vi "Top Level State Machine.vi"(8 "error in":errorcluster, 9 "Buses":T2[](array[typedef])=[{"Devices"=[{"Number of Channels"=1, "Device Alias"="", "Device Icon Name"=[]}], "Pin Information"={"List of IO Names"=["sbRIO-9651 Socket\\PMOD1_Pin4_out", "sbRIO-9651 Socket\\PMOD1_Pin3_in", "sbRIO-9651 Socket\\PMOD1_Pin2_out", "sbRIO-9651 Socket\\PMOD1_Pin1_out"], "List of Enable Lines"=["sbRIO-9651 Socket\\PMOD1_Pin4_enable", "sbRIO-9651 Socket\\PMOD1_Pin3_enable", "sbRIO-9651 Socket\\PMOD1_Pin2_enable", "sbRIO-9651 Socket\\PMOD1_Pin1_enable"]}, "Replacement VI for DLU"=path "E:/Documents/Projects/SPIAPI/Scripting Code  with State Machine 01_16_15 - Integrating with GUI/Test/Replacement.vi"}], 10 "Input Paths":T1={"Golden Template Directory"=path "E:/Documents/Projects/SPIAPI/Scripting Code  with State Machine 01_16_15 - Integrating with GUI/IONode", "Destination Directory"=path "E:/Documents/Projects/SPIAPI/Scripting Code  with State Machine 01_16_15 - Integrating with GUI/Test", "Destination Project"=path "E:/Documents/Projects/SPIAPI/Scripting Code  with State Machine 01_16_15 - Integrating with GUI/Test/Test.lvproj", "Destination VI"=path "E:/Documents/Projects/SPIAPI/Scripting Code  with State Machine 01_16_15 - Integrating with GUI/Test/TestVI.VI"}) -> (0 "error out":errorcluster)   [LabVIEW 2014, in "Initialization and IO Node Scripting.lvlib"]
uses:
  Initialization and IO Node Scripting.lvlib
  Scripting States.ctl
  Controls/Bus Information.ctl
  Controls/Device Information.ctl
  Controls/Pin Information.ctl
  Controls/Input Paths.ctl
  Controls/Values for Naming.ctl
  System.Windows.Forms
panel:
  out "Elapsed Time":dbl format="%<%H:%M:%S>t"
  in  "ProgressBar":refnum<k24>(container)
  in  "?":T5
  out "Status":string
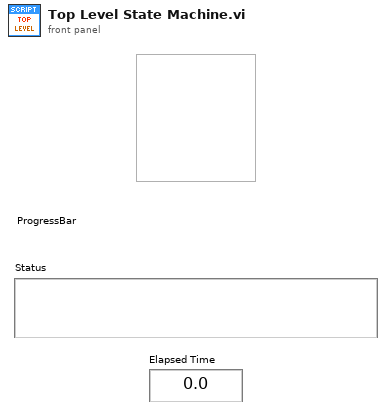
[diagram p1: front panel]
types:
  T1 = typedef "Input Paths.ctl" = cluster{"Golden Template Directory":path, "Destination Directory":path, "Destination Project":path, "Destination VI":path}
  T2 = typedef "Initialization and IO Node Scripting.lvlib/Bus Information.ctl" = cluster{"Devices":T3[], "Pin Information":T4, "Replacement VI for DLU":path}
  T3 = typedef "Device Information.ctl" = cluster{"Number of Channels":i32, "Device Alias":string, "Device Icon Name":string[]}
  T4 = typedef "Pin Information.ctl" = cluster{"List of IO Names":string[], "List of Enable Lines":string[]}
  T5 = typedef "Scripting States.ctl" = enum16{"Initialize", "Modify Dequeue Commands", "Modify Enqueue Data", "Create Project FIFOs", "Create and Place IO Nodes", "Update Node Count in Engine", "Expand FIFO Type Def", "Populate FIFO Names in Engine", "Modify I/O Pin Names", "Modify I/O Pin Enable", "Replace DLU", "Place SPI Engine", "Buses Complete Check", "End"}
  T6 = typedef "Initialization and IO Node Scripting.lvlib/Values for Naming.ctl" = cluster{"Bus Number":i32, "Device Number":i32, "Channel Number":i32}
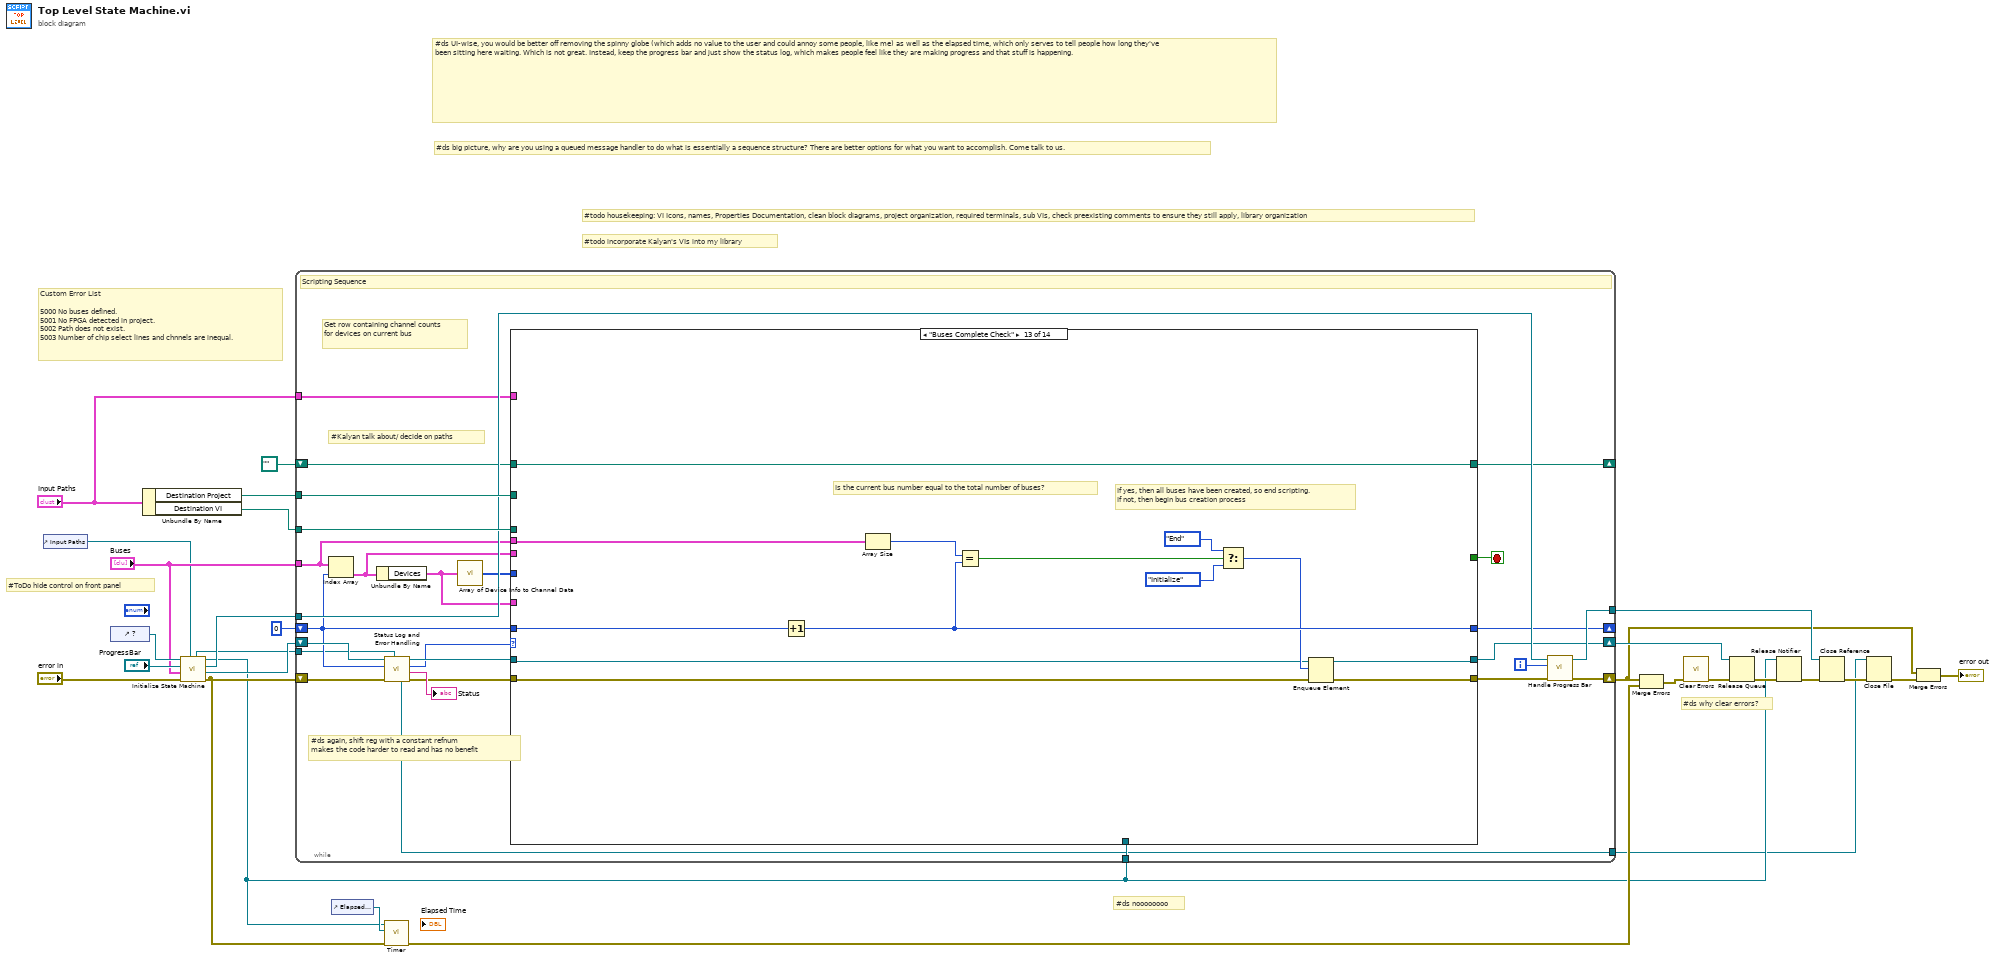
[diagram p0: block diagram]
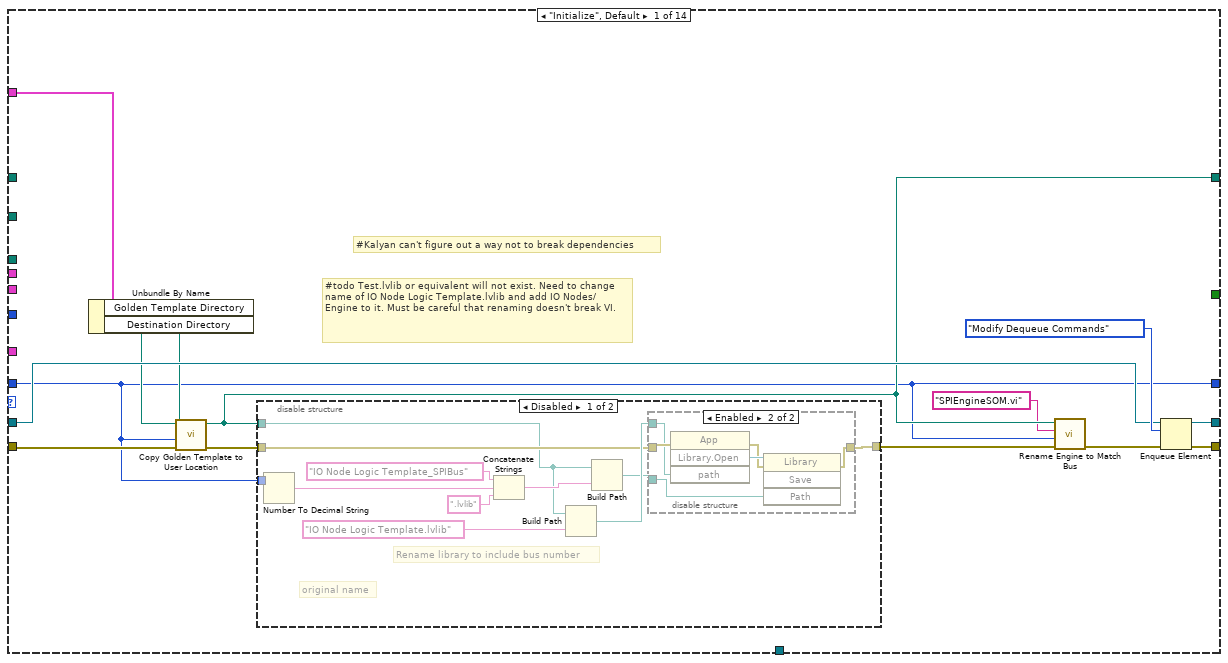
[diagram p2: hidden frame]
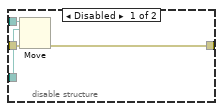
[diagram p3: hidden frame]
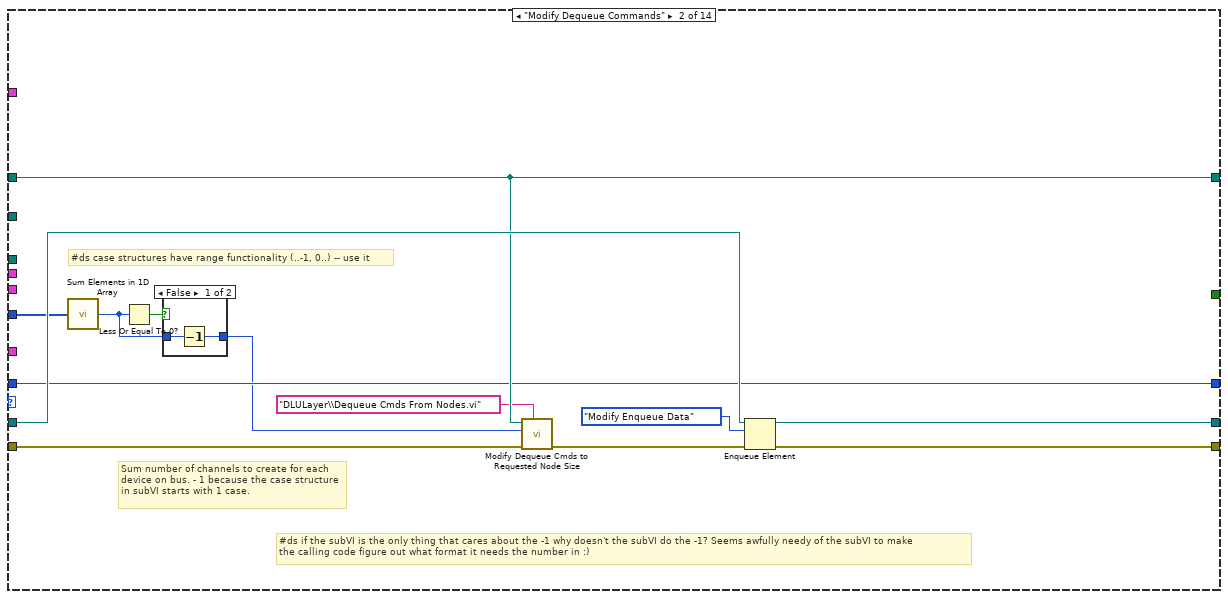
[diagram p5: hidden frame]
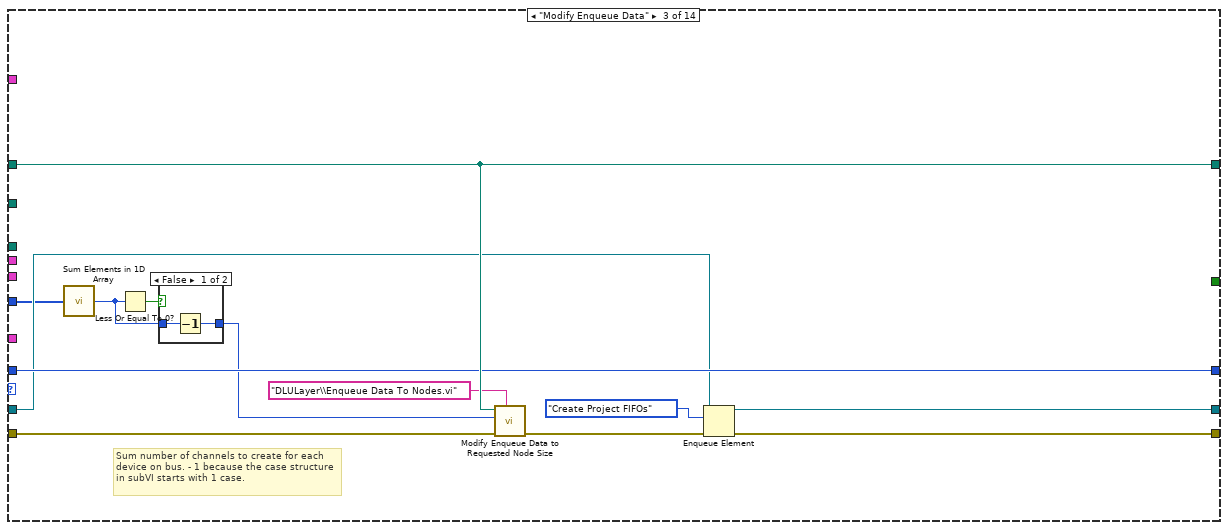
[diagram p7: hidden frame]
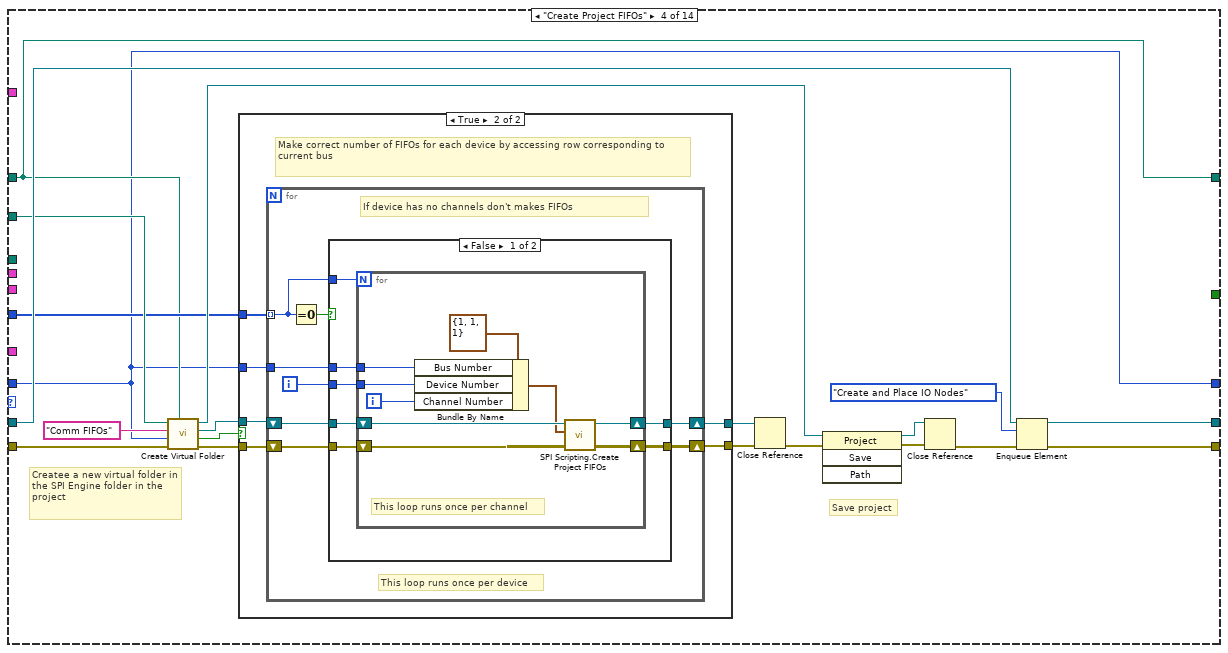
[diagram p9: hidden frame]
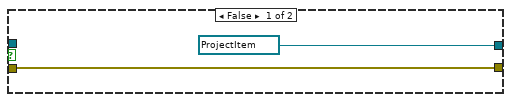
[diagram p10: hidden frame]
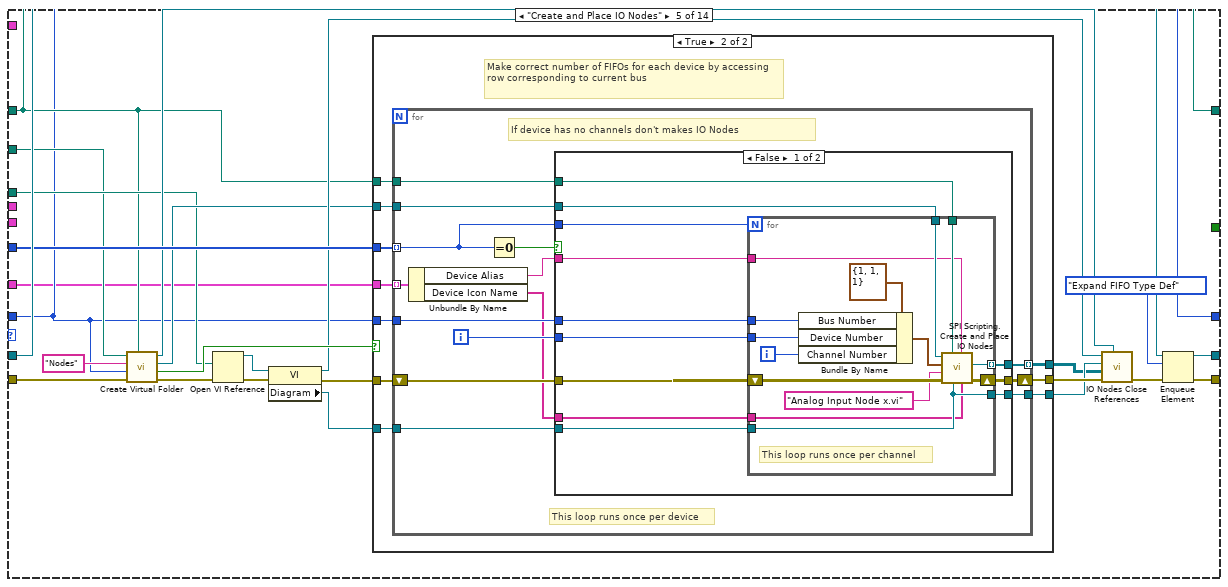
[diagram p12: hidden frame]
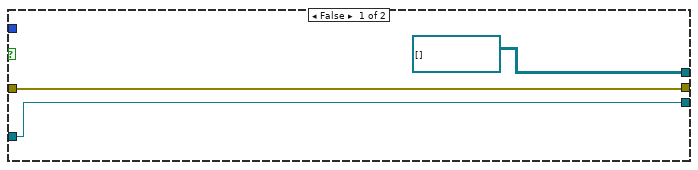
[diagram p13: hidden frame]
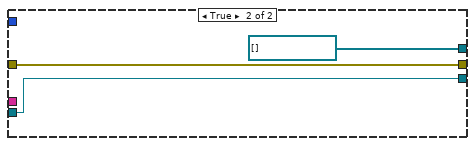
[diagram p14: hidden frame]
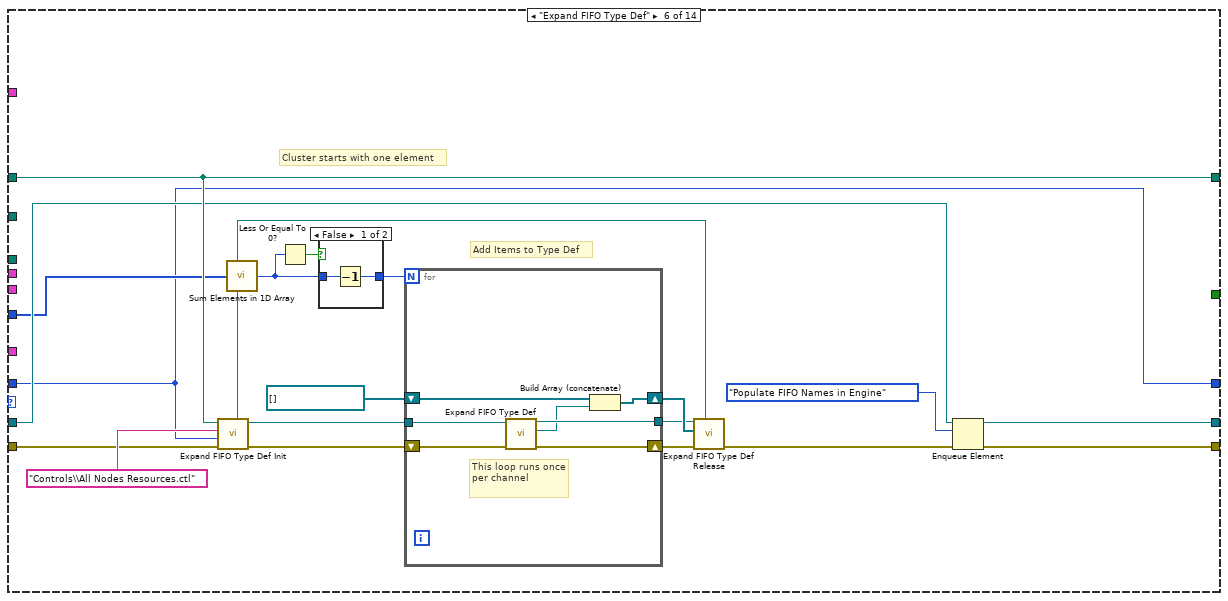
[diagram p15: hidden frame]
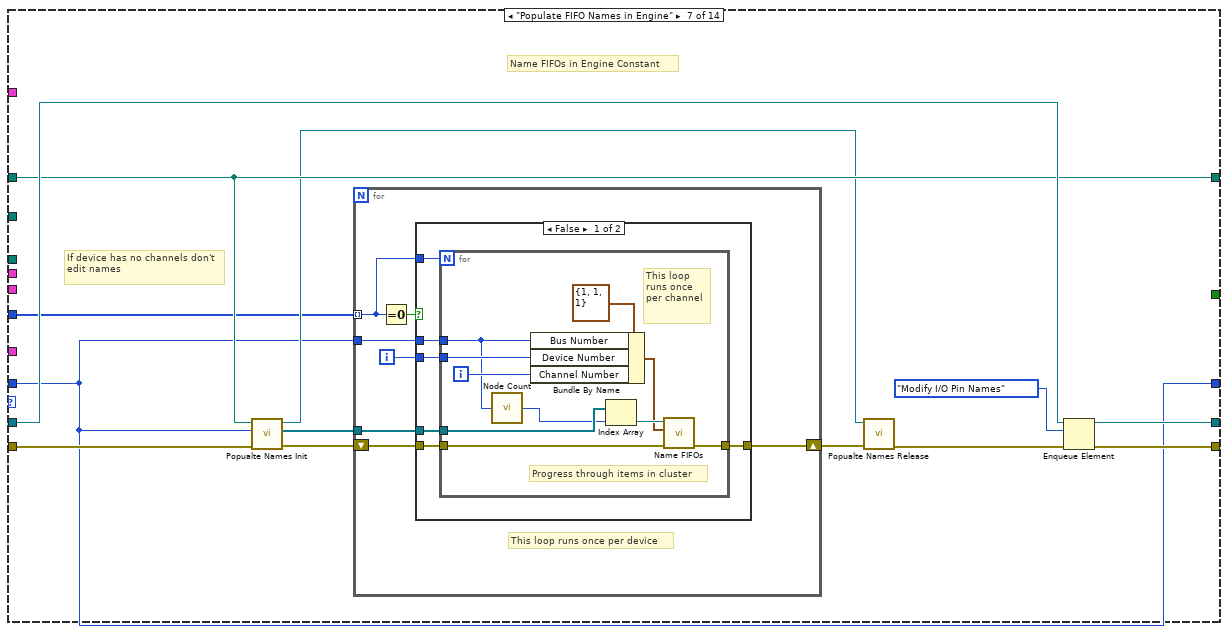
[diagram p17: hidden frame]
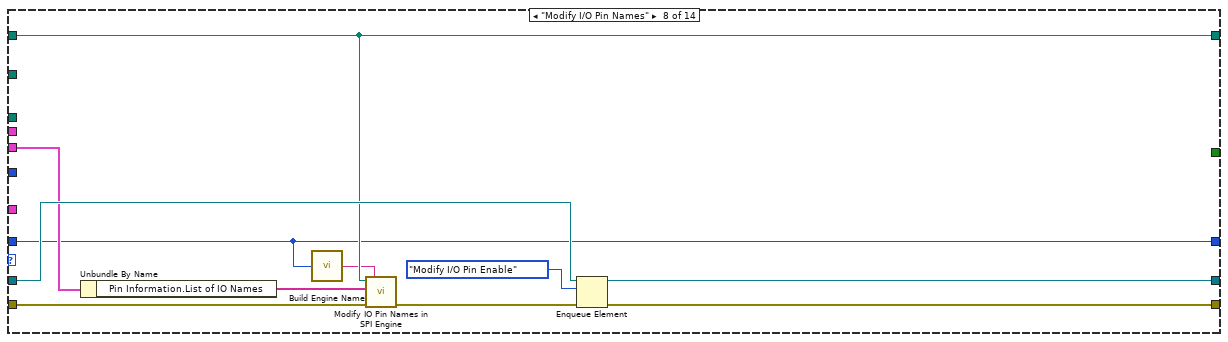
[diagram p19: hidden frame]
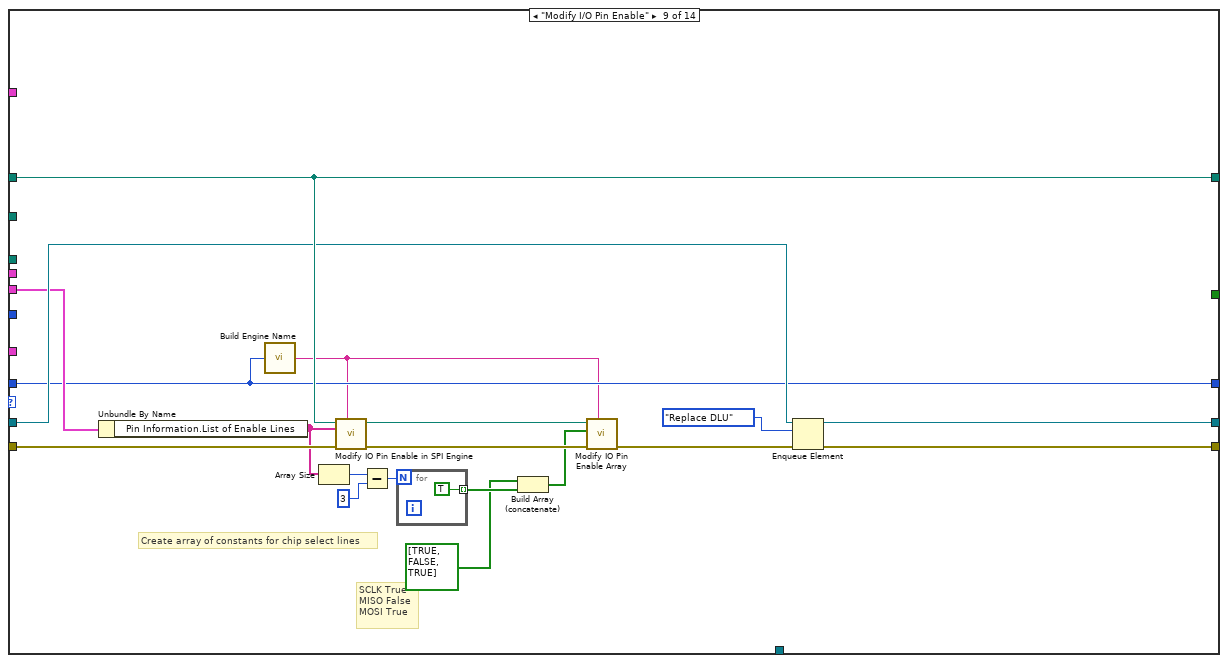
[diagram p20: hidden frame]
diagram:
  # "#ds big picture, why are you using a queued message handler to do what is essentially a sequence structure? There are better options for what you want to accomplish. Come talk to us."
  # "#ds why clear errors?"
  # "#ds noooooooo"
  # "#ds UI-wise, you would be better off removing the spinny globe (which adds no value to the user and could annoy some people, like me) as well as the elapsed time, which only serves to tell people how long they've been sitting here waiting. Which is not great. Instead, keep the progress bar and just show the status log, which makes people feel like they are making progress and that stuff is happening."
  # "Custom Error List\n\n5000 No buses defined.\n5001 No FPGA detected in project.\n5002 Path does not exist.\n5003 Number of chip select lines and chnnels are inequal."
  # "#todo incorporate Kalyan's VIs into my library"
  # "#todo housekeeping: VI Icons, names, Properties Documentation, clean block diagrams, project organization, required terminals, sub VIs, check preexisting comments to ensure they still apply, library organization"
  # "#ToDo hide control on front panel"
  n1 = control-ref of="Input Paths"() -> (w1:refnum<vi>)
  n2 = control-ref of="?"() -> (w16:refnum<vi>)
  n3 = Unbundle By Name("Input Paths") -> ("Destination Project"=w13:path, "Destination VI"=w12:path)
  n4 = call "Initialize State Machine.vi"("Input Paths Refnum"=w1, "error in (no error)"="error in", "Bus Info"="Buses", "ProgressBar in"="ProgressBar", "Enum Refnum"=w16) -> ("error out"=w26:errorcluster, "queue out"=w28:refnum<queue>, "ProgressBar out"=w22:refnum<k24>, "Notifier out"=w15:refnum<notifier>, "Status Log"=w3:refnum<file>)  [unwired: 2 in]
  n5 = while {
    shift-right: [w45] -> w9
    shift-left: w26 -> [w35]
    shift-right: [w46] -> w20
    shift-left: w28 -> [w37]
    tunnel: [w54] -> w23
    tunnel: w22 -> [w50]
    tunnel: w13 -> [w52]
    tunnel: w12 -> [w53]
    shift-right: [w49] -> _
    shift-left: 0 ("Number of SPI Buses") -> [w36]
    shift-right: [w48] -> _
    shift-left: path "" ("Curent Bus Path") -> [w47]
    tunnel: w15 -> [w43]
    tunnel: "Buses" -> [w42]
    tunnel: "Input Paths" -> [w40]
    tunnel: w3 -> [w30]
    tunnel: [w29] -> w2
    i -> [w51]
    stop <- w44 stop-if-true
    # "#ds again, shift reg with a constant refnum\nmakes the code harder to read and has no benefit"
    # "#Kalyan talk about/ decide on paths"
    # "Get row containing channel counts for devices on current bus"
    # "Scripting Sequence"
    n6 = Index Array(array=w42, index=w36) -> (element=w41:T2)
    n7 = Unbundle By Name(w41) -> ("Devices"=w38:T3[])
    n8 = call "Status Log and Error Handling.vi"("Status Log"=w30, "error in"=w35, "Current Bus Number"=w36, "Queue in"=w37) -> ("error out"=w31:errorcluster, "Current Status"=→"Status":string, "Next State"=w33:T5, "Queue out"=w34:refnum<queue>, "Status Log"=w29:refnum<file>)  [unwired: 3 in]
    n9 = call "Array of Device Info to Channel Data.vi"("Array of Devices"=w38) -> ("Device Channels"=w39:i32[])
    n10 = case shown="\"Buses Complete Check\"" w33 {
      tunnel: [w61 w92 w119 w142 w201 w268 w300 w335 w354 w365 w382 w399 w411 w422] -> w55
      tunnel: [w69 w104 w120 w143 w202 w267 w301 w336 w355 w366 w381 w400 w412 w427] -> w46
      tunnel: w31 -> [w67 w99 w115 w138 w194 w271 w291 w331 w352 w363 w377 w394 w413 w423]
      tunnel: w34 -> [w66 w102 w112 w140 w199 w266 w298 w333 w347 w364 w375 w396 w414 w427]
      tunnel: w47 -> [_ w100 w117 w125 w180 w270 w295 w330 w349 w361 w376 w391 w410 w430]
      tunnel: w52 -> [_ _ _ w137 w182 _ _ _ _ _ _ w384 _ _]
      tunnel: w53 -> [_ _ _ _ w183 _ _ _ _ _ _ w397 _ _]
      tunnel: w39 -> [_ w96 w109 w126 w198 w260 w290 _ _ _ w380 _ _ _]
      tunnel: w36 -> [w57 w98 w114 w124 w179 w259 w289 w327 w338 w360 w372 w392 w421 w431]
      tunnel: [w57 w98 w114 w124 w179 w259 w289 w327 w338 w360 w372 w392 w419 w431] -> w49
      tunnel: w42 -> [_ _ _ _ _ _ _ _ _ _ _ _ w418 _]
      tunnel: [w63 w100 w117 w125 w180 w270 w295 w330 w349 w361 w376 w391 w410 w430] -> w48
      tunnel: [_ _ _ _ _ _ _ _ _ _ _ _ _ TRUE] -> w44
      tunnel: w43 -> [_ _ _ _ _ _ _ _ _ _ _ _ _ w426]
      tunnel: w41 -> [_ _ _ _ _ _ _ w329 w343 w359 _ _ _ _]
      tunnel: w40 -> [w60 _ _ _ _ _ _ _ _ _ _ _ _ _]
      tunnel: w38 -> [_ _ _ _ w178 _ _ _ _ _ _ _ _ _]
      frame "Initialize", Default {
        # "#Kalyan can't figure out a way not to break dependencies"
        # "#todo Test.lvlib or equivalent will not exist. Need to change name of IO Node Logic Template.lvlib and add IO Nodes/ Engine to it. Must be careful that renaming doesn't break VI."
        n11 = Unbundle By Name(w60) -> ("Golden Template Directory"=w59:path, "Destination Directory"=w58:path)
        n12 = call "Copy Golden Template to User Location.vi"("Error In"=w67, "Bus Number"=w57, "Destination Path"=w58, "Golden Template Source Path"=w59) -> ("error out"=w64:errorcluster, "Curent Bus Path"=w63:path)  [unwired: 6 in]
        n13 = disable-structure shown="Disabled" {
          disable-tunnel: w64 -> [w74 w91]
          disable-tunnel: w57 -> [w73 _]
          disable-tunnel: w63 -> [w72 _]
          disable-tunnel: [w71 w91] -> w62
          frame Disabled {
            # "original name"
            # "Rename library to include bus number"
            n14 = Number To Decimal String(number=w73) -> (decimal integer string=w79:string)  [unwired: 1 in]
            n15 = Concatenate Strings("IO Node Logic Template_SPIBus" ("string"), w79, ".lvlib" ("string")) -> (w80:string)
            n16 = Build Path(base path=w72, name or relative path="IO Node Logic Template.lvlib" ("string")) -> (appended path=w76:path)
            n17 = Build Path(base path=w72, name or relative path=w80) -> (appended path=w75:path)
            n18 = disable-structure shown="Enabled" {
              disable-tunnel: w76 -> [w84 w86]
              disable-tunnel: w75 -> [w83 w85]
              disable-tunnel: w74 -> [w82 w87]
              disable-tunnel: [w81 w88] -> w71
              frame Disabled {
                n19 = Move(source path=w84, error in=w82, 10:w83) -> (error out=w81:errorcluster)  [unwired: 2 in, 2 out]
              }
              frame Enabled {
                n20 = invoke class="App" method="Library.Open"(error in=w87, "path"=w86) -> (error out=w89:errorcluster, "Open Library"=w90:refnum<vi>)  [unwired: 2 in, 2 out]
                n21 = invoke class="Library" method="Save"(reference=w90, error in=w89, "Path"=w85) -> (error out=w88:errorcluster)  [unwired: 1 in, 3 out]
              }
            }
          }
          frame Enabled {
          }
        }
        n22 = call "Rename Engine to Match Bus.vi"("error in (no error)"=w62, "Current Bus Number"=w57, "Path to File"="SPIEngineSOM.vi" ("Original File Name"), "Current Bus Path"=w63) -> ("error out"=w65:errorcluster)  [unwired: 6 in, 1 out]
        n23 = Enqueue Element(queue=w66, element=Scripting_States."Modify Dequeue Commands", error in (no error)=w65) -> (queue out=w69:refnum<queue>, error out=w61:errorcluster)  [unwired: 1 in, 1 out]
      }
      frame "Modify Dequeue Commands" {
        # "#ds if the subVI is the only thing that cares about the -1 why doesn't the subVI do the -1? Seems awfully needy of the subVI to make\nthe calling code figure out what format it needs the number in :)"
        # "#ds case structures have range functionality (..-1, 0..) -- use it"
        # "Sum number of channels to create for each device on bus. - 1 because the case structure in subVI starts with 1 case."
        n24 = call "Sum Elements in 1D Array.vi"("1D Array In"=w96) -> ("Sum of Elements"=w94:i32)
        n25 = Less Or Equal To 0?(x=w94) -> (x <= 0?=w95:bool)
        n26 = case shown="False" w95 {
          tunnel: w94 -> [w106 w107]
          tunnel: [w105 w107] -> w93
          frame False {
            n27 = Decrement(x=w106) -> (x-1=w105:i32)
          }
          frame True {
          }
        }
        n28 = call "Modify Dequeue Cmds to Requested Node Size.vi"("VI to Code Relative Path"="DLULayer\\Dequeue Cmds From Nodes.vi", "Error In"=w99, "NumCasesToAdd"=w93, "Source Root Path"=w100) -> ("Error Out"=w101:errorcluster)  [unwired: 5 in, 2 out]
        n29 = Enqueue Element(queue=w102, element=Scripting_States."Modify Enqueue Data", error in (no error)=w101) -> (queue out=w104:refnum<queue>, error out=w92:errorcluster)  [unwired: 1 in, 1 out]
      }
      frame "Modify Enqueue Data" {
        # "Sum number of channels to create for each device on bus. - 1 because the case structure in subVI starts with 1 case."
        n30 = call "Sum Elements in 1D Array.vi"("1D Array In"=w109) -> ("Sum of Elements"=w110:i32)
        n31 = Less Or Equal To 0?(x=w110) -> (x <= 0?=w111:bool)
        n32 = case shown="False" w111 {
          tunnel: w110 -> [w122 w123]
          tunnel: [w121 w123] -> w108
          frame False {
            n33 = Decrement(x=w122) -> (x-1=w121:i32)
          }
          frame True {
          }
        }
        n34 = call "Modify Enqueue Data to Requested Node Size.vi"("VI to Code Rel Path"="DLULayer\\Enqueue Data To Nodes.vi", "Error In"=w115, "NumCasesToAdd"=w108, "Source Root Path"=w117) -> ("error out"=w116:errorcluster)  [unwired: 5 in, 2 out]
        n35 = Enqueue Element(queue=w112, element=Scripting_States."Create Project FIFOs", error in (no error)=w116) -> (queue out=w120:refnum<queue>, error out=w119:errorcluster)  [unwired: 1 in, 1 out]
      }
      frame "Create Project FIFOs" {
        # "Save project"
        # "Createe a new virtual folder in the SPI Engine folder in the project"
        n36 = call "Create Virtual Folder.vi"("Curent Bus Path"=w125, "error in"=w138, "Bus Number"=w124, "Virtual Folder Name"="Comm FIFOs", "Path to Project"=w137) -> ("error out"=w130:errorcluster, "FPGA Target Found"=w128:bool, "New Virtual Folder"=w127:refnum<vi>, "Project:Open"=w131:refnum<vi>)  [unwired: 3 in]
        n37 = case shown="True" w128 {
          tunnel: [w145 w151] -> w132
          tunnel: w130 -> [w145 w150]
          tunnel: [refnum<vi> refnum ("Comm FIFOs Virtual Folder") w149] -> w129
          tunnel: w127 -> [_ w148]
          tunnel: w126 -> [_ w146]
          tunnel: w124 -> [_ w147]
          frame False {
          }
          frame True {
            # "Make correct number of FIFOs for each device by accessing row corresponding to current bus"
            n38 = for {
              shift-right: [w159] -> w151
              shift-left: w150 -> [w158]
              tunnel: w146 -> [w153] mode=indexing
              shift-right: [w157] -> w149
              shift-left: w148 -> [w156]
              tunnel: w147 -> [w152]
              i -> [w154]
              # "This loop runs once per device"
              # "If device has no channels don't makes FIFOs"
              n39 = Equal To 0?(x=w153) -> (x = 0?=w155:bool)
              n40 = case shown="False" w155 {
                tunnel: [w166 w177] -> w159
                tunnel: w158 -> [w165 w177]
                tunnel: [w164 w176] -> w157
                tunnel: w156 -> [w163 w176]
                tunnel: w154 -> [w162 _]
                tunnel: w153 -> [w161 _]
                tunnel: w152 -> [w160 _]
                frame False {
                  n41 = for {
                    N: w161 -> [_]
                    shift-right: [w175] -> w166
                    shift-left: w165 -> [w174]
                    shift-right: [w173] -> w164
                    shift-left: w163 -> [w172]
                    tunnel: w162 -> [w169]
                    tunnel: w160 -> [w168]
                    i -> [w170]
                    # "This loop runs once per channel"
                    n42 = Bundle By Name(cluster=T6 {"Bus Number"=1, "Device Number"=1, "Channel Number"=1} ("Values for Naming"), "Bus Number"=w168, "Device Number"=w169, "Channel Number"=w170) -> (w167:T6)
                    n43 = call "SPI Scripting.Create Project FIFOs.vi"("error in"=w174, "Values for Naming"=w167, "New Virtual Folder"=w172) -> ("error out"=w175:errorcluster, "Comm FIFOs Virtual Folder"=w173:refnum<vi>)  [unwired: 7 in]
                  }
                }
                frame True {
                }
              }
            }
          }
        }
        n44 = Close Reference(reference=w129, error in (no error)=w132) -> (error out=w136:errorcluster)
        n45 = invoke class="Project" method="Save"(reference=w131, error in=w136) -> (reference out=w134:refnum<vi>, error out=w135:errorcluster)  [unwired: 2 in, 2 out]
        n46 = Close Reference(reference=w134, error in (no error)=w135) -> (error out=w133:errorcluster)
        n47 = Enqueue Element(queue=w140, element=Scripting_States."Create and Place IO Nodes", error in (no error)=w133) -> (queue out=w143:refnum<queue>, error out=w142:errorcluster)  [unwired: 1 in, 1 out]
      }
      frame "Create and Place IO Nodes" {
        n48 = call "Create Virtual Folder.vi"("Curent Bus Path"=w180, "error in"=w194, "Bus Number"=w179, "Virtual Folder Name"="Nodes", "Path to Project"=w182) -> ("error out"=w193:errorcluster, "FPGA Target Found"=w191:bool, "New Virtual Folder"=w184:refnum<vi>, "Project:Open"=w188:refnum<vi>)  [unwired: 3 in]
        n49 = Open VI Reference(vi path=w183, error in (no error)=w193) -> (vi reference=w196:refnum<vi>, error out=w195:errorcluster)  [unwired: 4 in]
        n50 = property class="VI"(reference=w196, error in=w195) -> (reference out=w187:refnum<vi>, error out=w192:errorcluster, "Diagram"=w186:refnum<vi>)
        n51 = case shown="True" w191 {
          tunnel: [w204 w215] -> w190
          tunnel: w198 -> [_ w207]
          tunnel: w179 -> [_ w213]
          tunnel: w192 -> [w204 w214]
          tunnel: w186 -> [w205 w212]
          tunnel: [w205 w211] -> w185
          tunnel: w180 -> [_ w210]
          tunnel: w184 -> [_ w209]
          tunnel: [refnum<vi>[][] [] w208] -> w181
          tunnel: w178 -> [_ w206]
          frame False {
          }
          frame True {
            # "Make correct number of FIFOs for each device by accessing row corresponding to current bus"
            n52 = for {
              shift-right: [w229] -> w215
              shift-left: w214 -> [w228]
              tunnel: w207 -> [w225] mode=indexing
              tunnel: w213 -> [w224]
              tunnel: w212 -> [w223]
              tunnel: [w222] -> w211
              tunnel: w210 -> [w221]
              tunnel: w209 -> [w220]
              tunnel: [w219] -> w208 mode=indexing
              tunnel: w206 -> [w218] mode=indexing
              i -> [w226]
              # "This loop runs once per device"
              # "If device has no channels don't makes IO Nodes"
              n53 = Unbundle By Name(w218) -> ("Device Alias"=w217:string, "Device Icon Name"=w216:string[])
              n54 = Equal To 0?(x=w225) -> (x = 0?=w227:bool)
              n55 = case shown="False" w227 {
                tunnel: [w241 w258] -> w229
                tunnel: w228 -> [w240 w258]
                tunnel: w226 -> [w239 _]
                tunnel: w225 -> [w238 _]
                tunnel: w224 -> [w237 _]
                tunnel: w223 -> [w236 w257]
                tunnel: [w235 w257] -> w222
                tunnel: w221 -> [w234 _]
                tunnel: w220 -> [w233 _]
                tunnel: [w232 refnum<vi>[] []] -> w219
                tunnel: w217 -> [w231 _]
                tunnel: w216 -> [w230 _]
                frame False {
                  n56 = for {
                    N: w238 -> [_]
                    shift-right: [w254] -> w241
                    shift-left: w240 -> [w255]
                    tunnel: w239 -> [w250]
                    tunnel: w237 -> [w251]
                    tunnel: w236 -> [w253]
                    tunnel: [w253] -> w235
                    tunnel: w234 -> [w252]
                    tunnel: w233 -> [w247]
                    tunnel: [w246] -> w232 mode=indexing
                    tunnel: w231 -> [w242]
                    tunnel: w230 -> [w243]
                    i -> [w249]
                    # "This loop runs once per channel"
                    n57 = Bundle By Name(cluster=T6 {"Bus Number"=1, "Device Number"=1, "Channel Number"=1} ("Values for Naming"), "Bus Number"=w251, "Device Number"=w250, "Channel Number"=w249) -> (w245:T6)
                    n58 = call "SPI Scripting.Create and Place IO Nodes.vi"("Device Icon Name"=w243, "Device Alias"=w242, "Block Diagram"=w253, "Path to IO Node"=w252, "error in"=w255, "Path to Analog Node Template"="Analog Input Node x.vi", "Values for Naming"=w245, "Virtual Folder"=w247) -> ("error out"=w254:errorcluster, "New Copy of IO Node"=w246:refnum<vi>)  [unwired: 1 in, 1 out]
                  }
                }
                frame True {
                }
              }
            }
          }
        }
        n59 = call "IO Nodes Close References.vi"("Project in"=w188, "error in (no error)"=w190, "IO Nodes"=w181, "Diagram"=w185, "vi reference"=w187) -> ("error out"=w189:errorcluster)  [unwired: 6 in]
        n60 = Enqueue Element(queue=w199, element=Scripting_States."Expand FIFO Type Def", error in (no error)=w189) -> (queue out=w202:refnum<queue>, error out=w201:errorcluster)  [unwired: 1 in, 1 out]
      }
      frame "Expand FIFO Type Def" {
        # "Cluster starts with one element"
        # "Add Items to Type Def"
        n61 = call "Expand FIFO Type Def Init.vi"("error in (no error)"=w271, "Current Bus Number"=w259, "Path to All Nodes Resources"="Controls\\All Nodes Resources.ctl", "Destination Path"=w270) -> ("error out"=w274:errorcluster, "Cluster out"=w273:refnum<vi>, "Control Refnum"=w264:refnum<vi>)  [unwired: 5 in]
        n62 = call "Sum Elements in 1D Array.vi"("1D Array In"=w260) -> ("Sum of Elements"=w261:i32)
        n63 = Less Or Equal To 0?(x=w261) -> (x <= 0?=w262:bool)
        n64 = case shown="False" w262 {
          tunnel: w261 -> [w280 w281]
          tunnel: [w279 w281] -> w263
          frame False {
            n65 = Decrement(x=w280) -> (x-1=w279:i32)
          }
          frame True {
          }
        }
        n66 = for {
          N: w263 -> [_]
          shift-right: [w288] -> w275
          shift-left: w274 -> [w287]
          tunnel: w273 -> [w286]
          tunnel: [w285] -> w276
          shift-right: [w283] -> w277
          shift-left: refnum<vi>[] [] -> [w282]
          # "This loop runs once per channel"
          n67 = call "Expand FIFO Type Def.vi"("error in (no error)"=w287, "Cluster in"=w286) -> ("error out"=w288:errorcluster, "Clsuter Item"=w284:refnum<vi>, "Cluster out"=w285:refnum<vi>)  [unwired: 7 in]
          n68 = Build Array (concatenate)(w282, w284) -> (w283:refnum<vi>[])
        }
        n69 = call "Expand FIFO Type Def Release.vi"("Control Refnum"=w264, "error in (no error)"=w275, "Array"=w277, "Cluster in"=w276) -> ("error out"=w269:errorcluster)  [unwired: 7 in]
        n70 = Enqueue Element(queue=w266, element=Scripting_States."Populate FIFO Names in Engine", error in (no error)=w269) -> (queue out=w267:refnum<queue>, error out=w268:errorcluster)  [unwired: 1 in, 1 out]
      }
      frame "Populate FIFO Names in Engine" {
        # "If device has no channels don't edit names"
        # "Name FIFOs in Engine Constant"
        n71 = call "Popualte Names Init.vi"("error in (no error)"=w291, "Current Bus Number"=w289, "Destination Path"=w295) -> ("error out"=w297:errorcluster, "Communication FIFOs Elements"=w292:refnum<vi>[], "Communication FIFOs Refnum"=w294:refnum<vi>)  [unwired: 6 in]
        n72 = for {
          tunnel: w292 -> [w306]
          shift-right: [w307] -> w296
          shift-left: w297 -> [w308]
          tunnel: w290 -> [w302] mode=indexing
          tunnel: w289 -> [w303]
          i -> [w305]
          # "This loop runs once per device"
          n73 = Equal To 0?(x=w302) -> (x = 0?=w304:bool)
          n74 = case shown="False" w304 {
            tunnel: w308 -> [w314 w325]
            tunnel: [w313 w325] -> w307
            tunnel: w306 -> [w312 _]
            tunnel: w305 -> [w311 _]
            tunnel: w302 -> [w310 _]
            tunnel: w303 -> [w309 _]
            frame False {
              n75 = for {
                N: w310 -> [_]
                tunnel: [w324] -> w313
                tunnel: w314 -> [w323]
                tunnel: w312 -> [w322]
                tunnel: w311 -> [w318]
                tunnel: w309 -> [w316]
                i -> [w317]
                # "This loop runs once per channel"
                # "Progress through items in cluster"
                n76 = call "Node Count.vi"("Bus Number in"=w316) -> ("Node Number"=w315:i32)
                n77 = Bundle By Name(cluster=T6 {"Bus Number"=1, "Device Number"=1, "Channel Number"=1} ("Values for Naming"), "Bus Number"=w316, "Device Number"=w318, "Channel Number"=w317) -> (w320:T6)
                n78 = Index Array(array=w322, index=w315) -> (element=w321:refnum<vi>)
                n79 = call "Name FIFOs.vi"("error in (no error)"=w323, "Values for Naming"=w320, "Communications FIFOs Element"=w321) -> ("error out"=w324:errorcluster)  [unwired: 8 in]
              }
            }
            frame True {
            }
          }
        }
        n80 = call "Popualte Names Release.vi"("error in (no error)"=w296, "ClusterConstant in"=w294) -> ("error out"=w293:errorcluster)  [unwired: 9 in]
        n81 = Enqueue Element(queue=w298, element=Scripting_States."Modify I/O Pin Names", error in (no error)=w293) -> (queue out=w301:refnum<queue>, error out=w300:errorcluster)  [unwired: 1 in, 1 out]
      }
      frame "Modify I/O Pin Names" {
        n82 = Unbundle By Name(w329) -> ("Pin Information.List of IO Names"=w328:string[])
        n83 = call "Build Engine Name.vi"("Current Bus Number"=w327) -> ("Engine Name"=w326:string)
        n84 = call "Modify IO Pin Names in SPI Engine.vi"("VI to Code Relative Path"=w326, "Error In"=w331, "List of IO Names"=w328, "Source Root Path"=w330) -> ("Error Out"=w332:errorcluster)  [unwired: 5 in, 2 out]
        n85 = Enqueue Element(queue=w333, element=Scripting_States."Modify I/O Pin Enable", error in (no error)=w332) -> (queue out=w336:refnum<queue>, error out=w335:errorcluster)  [unwired: 1 in, 1 out]
      }
      frame "Modify I/O Pin Enable" {
        # "Create array of constants for chip select lines"
        # "SCLK True\nMISO False\nMOSI True"
        n86 = Unbundle By Name(w343) -> ("Pin Information.List of Enable Lines"=w342:string[])
        n87 = call "Build Engine Name.vi"("Current Bus Number"=w338) -> ("Engine Name"=w337:string)
        n88 = Array Size(array=w342) -> (size(s)=w340:i32)
        n89 = call "Modify IO Pin Enable in SPI Engine.vi"("VI to Code Relative Path"=w337, "Error In"=w352, "List of Enable Lines"=w342, "Source Root Path"=w349) -> ("Error Out"=w351:errorcluster, "Source Root Path Out"=w348:path)  [unwired: 5 in, 1 out]
        n90 = Subtract(x=w340, y=3) -> (x-y=w341:i32)
        n91 = for {
          N: w341 -> [_]
          tunnel: [TRUE] -> w346 mode=indexing
        }
        n92 = Build Array (concatenate)(bool[] [TRUE, FALSE, TRUE], w346) -> (w344:bool[])
        n93 = call "Modify IO Pin Enable Array.vi"("VI to Code Relative Path"=w337, "Error In"=w351, "Enable"=w344, "Source Root Path"=w348) -> ("Error Out"=w350:errorcluster)  [unwired: 5 in, 2 out]
        n94 = Enqueue Element(queue=w347, element=Scripting_States."Replace DLU", error in (no error)=w350) -> (queue out=w355:refnum<queue>, error out=w354:errorcluster)  [unwired: 1 in, 1 out]
      }
      frame "Replace DLU" {
        n95 = Unbundle By Name(w359) -> ("Replacement VI for DLU"=w358:path)
        n96 = call <vilib>:"Is Path and Not Empty.vi"("path"=w358) -> ("Is Path and Not Empty?"=w357:bool)  [unwired: 4 in]
        n97 = case shown="True" w357 {
          tunnel: w363 -> [w368 w371]
          tunnel: [w368 w370] -> w362
          tunnel: w361 -> [_ w369]
          frame False {
          }
          frame True {
            n98 = call "Replace DLU.vi"("error in"=w371, "Current Bus Path"=w369) -> ("error out"=w370:errorcluster)  [unwired: 9 in]
          }
        }
        n99 = Enqueue Element(queue=w364, element=Scripting_States."Update Node Count in Engine", error in (no error)=w362) -> (queue out=w366:refnum<queue>, error out=w365:errorcluster)  [unwired: 1 in, 1 out]
      }
      frame "Update Node Count in Engine" {
        n100 = call "Sum Elements in 1D Array.vi"("1D Array In"=w380) -> ("Sum of Elements"=w379:i32)
        n101 = call "Build Engine Name.vi"("Current Bus Number"=w372) -> ("Engine Name"=w373:string)
        n102 = call "Modify NumNodes in SPI Engine.vi"("VI to Code Relative Path"=w373, "Error In"=w377, "Number of Nodes"=w379, "Source Root Path"=w376) -> ("Error Out"=w378:errorcluster)  [unwired: 4 in, 3 out]
        n103 = Enqueue Element(queue=w375, element=Scripting_States."Place SPI Engine", error in (no error)=w378) -> (queue out=w381:refnum<queue>, error out=w382:errorcluster)  [unwired: 1 in, 1 out]
      }
      frame "Place SPI Engine" {
        # "If FPGA target not found, don't execute"
        n104 = call "Create Virtual Folder.vi"("Curent Bus Path"=w391, "error in"=w394, "Bus Number"=w392, "Virtual Folder Name"="Engine", "Path to Project"=w384) -> ("error out"=w393:errorcluster, "FPGA Target Found"=w385:bool, "New Virtual Folder"=w386:refnum<vi>, "Project:Open"=w387:refnum<vi>)  [unwired: 3 in]
        n105 = case shown="True" w385 {
          tunnel: w397 -> [_ w408]
          tunnel: w393 -> [w401 w407]
          tunnel: w392 -> [_ w402]
          tunnel: w391 -> [_ w406]
          tunnel: [w401 w405] -> w383
          tunnel: w386 -> [_ w404]
          frame False {
          }
          frame True {
            n106 = call "Build Engine Name.vi"("Current Bus Number"=w402) -> ("Engine Name"=w403:string)
            n107 = call "SPI Scripting.SPI Engine.vi"("SPI Engine Name"=w403, "Path to Place SPI Engine"=w408, "error in"=w407, "Bus Number"=w402, "New Virtual Folder"=w404, "Path to IO Node"=w406) -> ("error out"=w405:errorcluster)  [unwired: 4 in, 1 out]
          }
        }
        n108 = invoke class="Project" method="Save"(reference=w387, error in=w383, "Path"=w384) -> (reference out=w389:refnum<vi>, error out=w390:errorcluster)  [unwired: 1 in, 2 out]
        n109 = Close Reference(reference=w389, error in (no error)=w390) -> (error out=w388:errorcluster)
        n110 = Enqueue Element(queue=w396, element=Scripting_States."Buses Complete Check", error in (no error)=w388) -> (queue out=w400:refnum<queue>, error out=w399:errorcluster)  [unwired: 1 in, 1 out]
      }
      frame "Buses Complete Check" {
        # "If yes, then all buses have been created, so end scripting.\nIf not, then begin bus creation process"
        # "Is the current bus number equal to the total number of buses?"
        n111 = Increment(x=w421) -> (x+1=w419:i32)
        n112 = Array Size(array=w418) -> (size(s)=w409:i32)
        n113 = Equal?(x=w409, y=w419) -> (x = y?=w420:bool)
        n114 = Select(t=Scripting_States."End", s=w420, f=Scripting_States."Initialize") -> (s? t:f=w415:T5)
        n115 = Enqueue Element(queue=w414, element=w415, error in (no error)=w413) -> (queue out=w412:refnum<queue>, error out=w411:errorcluster)  [unwired: 1 in, 1 out]
      }
      frame "End" {
        # "Stop Timer"
        n116 = call <vilib>:"Clear Errors.vi"("error in (no error)"=w423) -> ("error out"=w425:errorcluster)  [unwired: 5 in, 1 out]
        n117 = Send Notification(notification=TRUE, notifier=w426, error in (no error)=w425) -> (error out=w424:errorcluster)  [unwired: 1 out]
        n118 = Merge Errors(w423, w424) -> (w422:errorcluster)
      }
    }
    n119 = call "Handle Progress Bar.vi"("error in"=w55, "Numeric"=w51, ".NET Refnum in"=w50) -> ("error out"=w45:errorcluster, ".NET Refnum out"=w54:refnum<k24>)  [unwired: 7 in]
  }
  n120 = control-ref of="Elapsed Time"() -> (w17:refnum<vi>)
  n121 = call "Timer.vi"("error in (no error)"=w26, "DigNum Refnum"=w17, "Notifier in"=w15) -> ("error out"=w21:errorcluster)  [unwired: 8 in]
  n122 = Merge Errors(w9, w21) -> (w7:errorcluster)
  n123 = call <vilib>:"Clear Errors.vi"("error in (no error)"=w7) -> ("error out"=w8:errorcluster)  [unwired: 5 in, 1 out]
  n124 = Release Queue(queue=w20, error in (no error)=w8) -> (error out=w25:errorcluster)  [unwired: 1 in, 2 out]
  n125 = Release Notifier(notifier=w15, error in (no error)=w25) -> (error out=w24:errorcluster)  [unwired: 1 in, 2 out]
  n126 = Close Reference(reference=w23, error in (no error)=w24) -> (error out=w6:errorcluster)
  n127 = Close File(refnum=w2, error in=w6) -> (error out=w5:errorcluster)  [unwired: 1 out]
  n128 = Merge Errors(w9, w5) -> (→"error out":errorcluster)
